vi "Stream With Replicate.vi"() -> ()   [LabVIEW 2023]
doc: "This VI demonstrates use of the Stream with replication, a channel wire that communicates data among parallel loops and easily handling many of the complex scenarios for managing the controlled shutdown of that connection."
uses:
  <extravilib>/ChannelInstances/Stream-i32/Endpoint.vi
  <extravilib>/ChannelInstances/Stream-i32/EndpointRead.vi
  <extravilib>/ChannelInstances/Stream-i32/Instantiate.vi
  <extravilib>/ChannelInstances/Stream-i32/)Channel.vi
  <resource>/ChannelSupport/_ChannelSupport/WaitIfNeeded.vi
  <extravilib>/ChannelInstances/Stream-i32.lvlib
panel:
  in  "Independent Abort?":bool
  in  "Delay 1":u32=50
  in  "Delay 2":u32=100
  in  "Stop Consumer 2":bool
  out "Data Consumed 2":i32(graph)
  in  "Consumer Stop Value 2":i32=-1
  in  "Consumer Stop Value":i32=-1
  in  "Emergency Stop Producer":bool
  out "Data Consumed":i32(graph)
  out "Data Produced":i32(graph)
  in  "Stop Consumer":bool
  in  "Stop Producer":bool
  # "Overview: This VI assumes you have already looked at the other VI in this project: Stream.vi.\nThis VI shows the use of the Replicate function. A single Stream goes in and two such Streams come out. The content of the original stream is duplicated so that both of the output streams get their own copy of the data. The consumers of the replicated streams start off consuming the data at different rates. This example lets you see the effects of different rates of consumption on the system overall. Notice that with a bounded buffer, the consumer loops will tend to synchronize because data can only be replicated at the rate of the slowest consumer loop.\nInstructions:\n1. Configure the two Delay values for the two consumer loops. Select whether the loops have independent abort or not.\n2. Run the VI. Press the Normal Stop Producer button to see the producer stop; the consumers both continue until they each catch up.\n3. Run the VI again. The Emergency Stop Producer button will halt all the consumers as quickly as possible.\n4. Run the VI again. Any of the other stop conditions depend upon the \"Independent Abort?\" setting. If it is false then the two replicas share an abort signal: aborting one for any reason will abort the other. If it is true then one replica can stop but the producer will continue producing data for the other one."
  # "Set These Before Running VI"
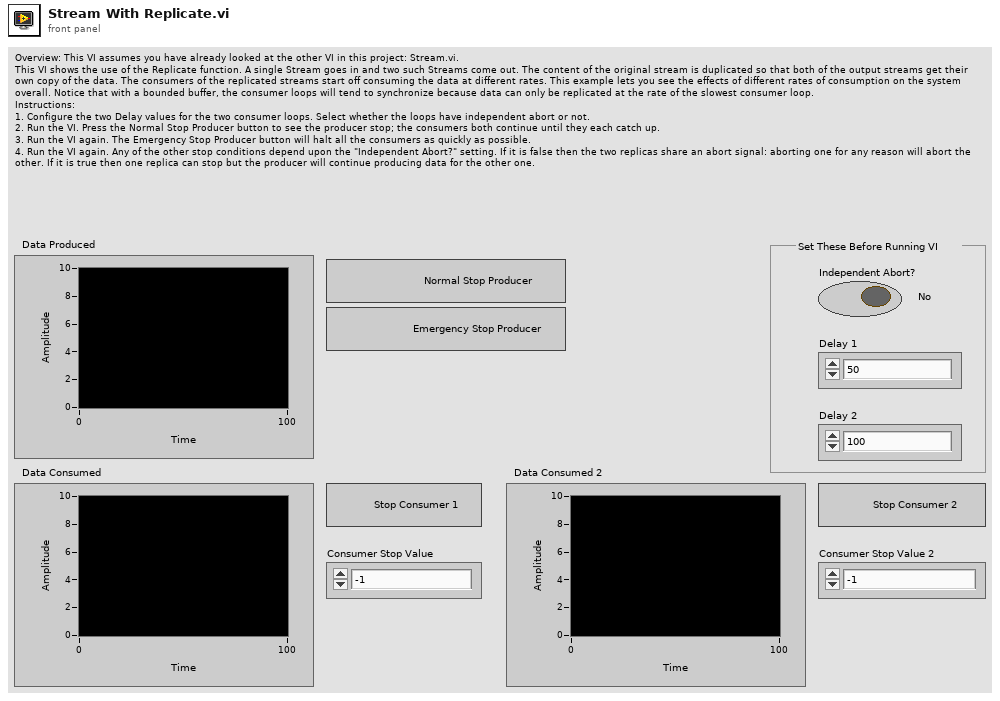
[diagram p1: front panel]
types:
  T1 = typedef "Stream-i32.lvlib/)Channel.ctl" = refnum<queue>
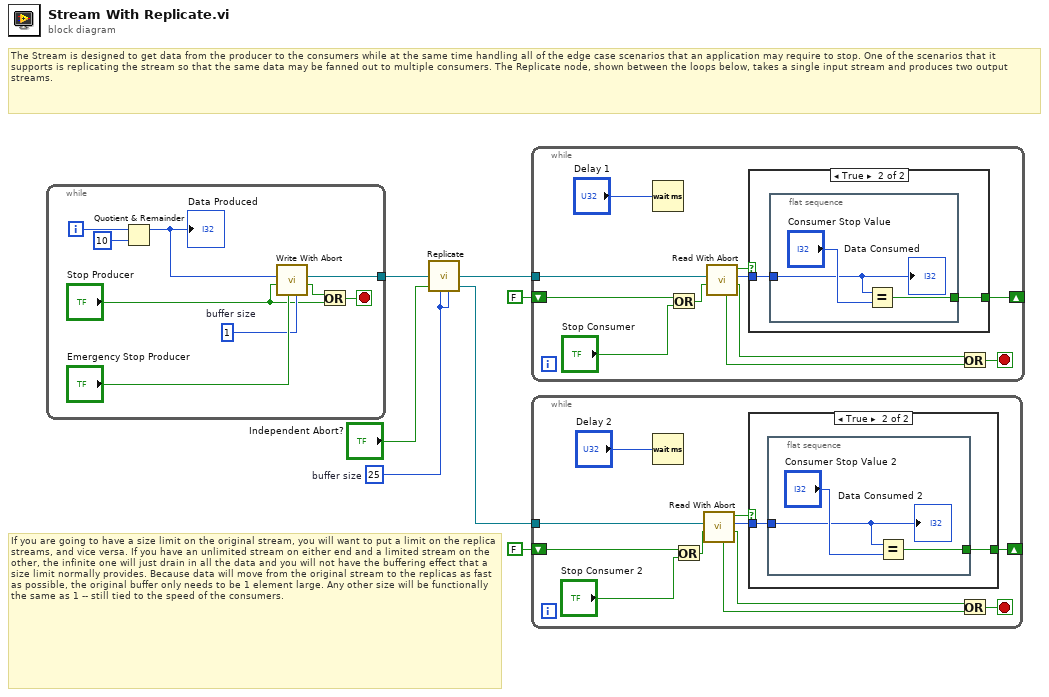
[diagram p0: block diagram]
diagram:
  w1 = 25  # buffer size
  # "If you are going to have a size limit on the original stream, you will want to put a limit on the replica streams, and vice versa. If you have an unlimited stream on either end and a limited stream on the other, the infinite one will just drain in all the data and you will not have the buffering effect that a size limit normally provides. Because data will move from the original stream to the replicas as fast as possible, the original buffer only needs to be 1 element large. Any other size will be functionally the same as 1 -- still tied to the speed of the consumers."
  # "The Stream is designed to get data from the producer to the consumers while at the same time handling all of the edge case scenarios that an application may require to stop. One of the scenarios that it supports is replicating the stream so that the same data may be fanned out to multiple consumers. The Replicate node, shown between the loops below, takes a single input stream and produces two output streams."
  n1 = while {
    tunnel: [w13] -> w7
    i -> [w15]
    stop <- w10 stop-if-true
    w11 = 1  # buffer size
    n2 = Quotient & Remainder(x=w15, y=10) -> (x-y*floor(x/y)=w14:i32)  [unwired: 1 out]
    "Data Produced" <- w14
    n3 = call <extravilib>:"Write With Abort.vi"("size (unlimited)"=w11, "abort"="Emergency Stop Producer", "last element? (F)"="Stop Producer", "element"=w14) -> ("aborted?"=w9:bool, "channel"=w13:T1)  [unwired: 4 in, 2 out]
    n4 = Or(x=w9, y="Stop Producer") -> (x .or. y?=w10:bool)
  }
  n5 = call <extravilib>:"Replicate.vi"("stream"=w7, "independent aborts? (F)"="Independent Abort?", "copy 1 size (unlimited)"=w1, "copy 2 size (unlimited)"=w1) -> ("stream copy 1"=w6:T1, "stream copy 2"=w5:T1)  [unwired: 4 in]
  n6 = while {
    tunnel: w6 -> [w25]
    shift-right: [w18] -> _
    shift-left: FALSE -> [w17]
    stop <- w27 stop-if-true
    n7 = Wait (ms)(milliseconds to wait="Delay 1") -> ()  [unwired: 1 out]
    n8 = Or(x=w17, y="Stop Consumer") -> (x .or. y?=w20:bool)
    n9 = call <extravilib>:"Read With Abort.vi"("abort"=w20, "channel"=w25) -> ("last element?"=w22:bool, "element"=w24:i32, "element valid?"=w23:bool, "aborted?"=w19:bool)  [unwired: 4 in, 2 out]
    n10 = case shown="True" w23 {
      tunnel: w24 -> [_ w29]
      tunnel: [_ w28] -> w18
      frame False {
      }
      frame True {
        n11 = flat-sequence {
          tunnel: w29 -> [w31]
          tunnel: [w30] -> w28
          frame #0 {
            n12 = Equal?(x=w31, y="Consumer Stop Value") -> (x = y?=w30:bool)
            "Data Consumed" <- w31
          }
        }
      }
    }
    n13 = Or(x=w22, y=w19) -> (x .or. y?=w27:bool)
  }
  n14 = while {
    tunnel: w5 -> [w41]
    shift-right: [w34] -> _
    shift-left: FALSE -> [w33]
    stop <- w43 stop-if-true
    n15 = Wait (ms)(milliseconds to wait="Delay 2") -> ()  [unwired: 1 out]
    n16 = Or(x=w33, y="Stop Consumer 2") -> (x .or. y?=w37:bool)
    n17 = call <extravilib>:"Read With Abort.vi"("abort"=w37, "channel"=w41) -> ("last element?"=w38:bool, "element"=w40:i32, "element valid?"=w39:bool, "aborted?"=w35:bool)  [unwired: 4 in, 2 out]
    n18 = case shown="True" w39 {
      tunnel: w40 -> [_ w45]
      tunnel: [_ w44] -> w34
      frame False {
      }
      frame True {
        n19 = flat-sequence {
          tunnel: w45 -> [w47]
          tunnel: [w46] -> w44
          frame #0 {
            n20 = Equal?(x=w47, y="Consumer Stop Value 2") -> (x = y?=w46:bool)
            "Data Consumed 2" <- w47
          }
        }
      }
    }
    n21 = Or(x=w38, y=w35) -> (x .or. y?=w43:bool)
  }
